vi "Pick modules.vi"(1 "Module List":T1(array[cluster])=[{"Enable"=TRUE, "Abs Start Time"=1500.0, "Module"=34, "String"="", "Array"=[]}, {"Enable"=FALSE, "Abs Start Time"=2000.0, "Module"=0, "String"="", "Array"=[]}, {"Enable"=FALSE, "Abs Start Time"=3000.0, "Module"=0, "String"="", "Array"=[]}, {"Enable"=FALSE, "Abs Start Time"=4000.0, "Module"=0, "String"="", "Array"=[]}, {"Enable"=TRUE, "Abs Start Time"=8000.0, "Module"=4, "String"="", "Array"=[]}, {"Enable"=FALSE, "Abs Start Time"=6000.0, "Module"=0, "String"="", "Array"=[]}] {"Module" items=["Atom removal 1", "Atom removal 2", "B-field off", "CMOT", "Defaults", "Final B-field ramps", "Fluorescence pulse", "High field", "High field ARP", "Loading cart QT", "Loading sci QT", "Low field", "Low field ARP", "Mol OD image", "Mol picture", "Mol probe pulse", "Molasses", "MOT off", "MOT on", "OD image", "Optical pumping", "OT B-field off", "Picture", "Probe pulse", "QT off for OT", "Quadrupole trap off", "Quadrupole trap", "Quantization axis", "S-G separation", "STIRAP back for imaging", "STIRAP", "TTL high", "TTL low", "GPIB", "Utility Module 1", "Utility Module 2", "Utility Module 3", "Utility Module 4", "Utility Module 5", "Utility Module 6", "Utility Module 7", "Utility Module 8", "Utility Module 9"]; "Abs Start Time" format="%.3f"}) -> (2 "Output Data":i64[][](array[numeric])=[[1600000, 3, 31, 1], [1600001, 3, 31, 0], [1700000, 3, 31, 1], [1700001, 3, 31, 0], [1800000, 3, 31, 1], [1800001, 3, 31, 0], [8000000, 0, 0, 0], [8000000, 0, 1, 0], [8000000, 0, 2, 0], [8000000, 0, 3, 0], [8000000, 0, 4, 1], [8000000, 0, 5, 0], [8000000, 0, 6, 0], [8000000, 0, 7, 0], [8000000, 0, 8, 0], [8000000, 0, 9, 1], [8000000, 0, 10, 0], [8000000, 0, 11, 0], [8000000, 0, 12, 0], [8000000, 0, 13, 0], [8000000, 0, 14, 1], [8000000, 0, 15, 0], [8000000, 0, 16, 0], [8000000, 0, 17, 0], [8000000, 0, 18, 0], [8000000, 0, 19, 1], [8000000, 0, 20, 0], [8000000, 0, 21, 0], [8000000, 0, 22, 0], [8000000, 0, 23, 0], [8000000, 0, 24, 1], [8000000, 0, 25, 0], [8000000, 0, 26, 0], [8000000, 0, 27, 0], [8000000, 0, 28, 0], [8000000, 0, 29, 0], [8000000, 0, 30, 0], [8000000, 0, 31, 0], [8000000, 1, 0, 0], [8000000, 1, 1, 0], [8000000, 1, 2, 0], [8000000, 1, 3, 0], [8000000, 1, 4, 0], [8000000, 1, 5, 0], [8000000, 1, 6, 0], [8000000, 1, 7, 0], [8000000, 1, 8, 0], [8000000, 1, 9, 0], [8000000, 1, 10, 0], [8000000, 1, 11, 0], [8000000, 1, 12, 0], [8000000, 1, 13, 0], [8000000, 1, 14, 0], [8000000, 1, 15, 0], [8000000, 1, 16, 0], [8000000, 1, 17, 1], [8000000, 1, 18, 0], [8000000, 1, 19, 0], [8000000, 1, 20, 0], [8000000, 1, 21, 0], [8000000, 1, 22, 0], [8000000, 1, 23, 0], [8000000, 1, 24, 0], [8000000, 1, 25, 0], [8000000, 1, 26, 0], [8000000, 1, 27, 0], [8000000, 1, 28, 0], [8000000, 1, 29, 0], [8000000, 1, 30, 0], [8000000, 1, 31, 0], [8000000, 2, 0, 0], [8000000, 2, 1, 0], [8000000, 2, 2, 0], [8000000, 2, 3, 0], [8000000, 2, 4, 0], [8000000, 2, 5, 0], [8000000, 2, 6, 0], [8000000, 2, 7, 0], [8000000, 2, 8, 0], [8000000, 2, 9, 0], [8000000, 2, 10, 0], [8000000, 2, 11, 0], [8000000, 2, 12, 0], [8000000, 2, 13, 0], [8000000, 2, 14, 0], [8000000, 2, 15, 0], [8000000, 2, 16, 0], [8000000, 2, 17, 0], [8000000, 2, 18, 0], [8000000, 2, 19, 0], [8000000, 2, 20, 0], [8000000, 2, 21, 0], [8000000, 2, 22, 0], [8000000, 2, 23, 0], [8000000, 2, 24, 0], [8000000, 2, 25, 0], [8000000, 2, 26, 0], [8000000, 2, 27, 0], [8000000, 2, 28, 0], [8000000, 2, 29, 0], [8000000, 2, 30, 0], [8000000, 2, 31, 0], [8000000, 3, 0, 0], [8000000, 3, 1, 0], [8000000, 3, 2, 0], [8000000, 3, 3, 0], [8000000, 3, 4, 0], [8000000, 3, 5, 0], [8000000, 3, 6, 0], [8000000, 3, 7, 0], [8000000, 3, 8, 0], [8000000, 3, 9, 0], [8000000, 3, 10, 0], [8000000, 3, 11, 0], [8000000, 3, 12, 0], [8000000, 3, 13, 0], [8000000, 3, 14, 0], [8000000, 3, 15, 0], [8000000, 3, 16, 0], [8000000, 3, 17, 0], [8000000, 3, 18, 0], [8000000, 3, 19, 0], [8000000, 3, 20, 0], [8000000, 3, 21, 0], [8000000, 3, 22, 0], [8000000, 3, 23, 0], [8000000, 3, 24, 0], [8000000, 3, 25, 0], [8000000, 3, 26, 0], [8000000, 3, 27, 0], [8000000, 3, 28, 0], [8000000, 3, 29, 0], [8000000, 3, 30, 0], [8000000, 3, 31, 0]], 3 "GPIB output":T1(array[cluster]) {"Module" items=["TTL high                                                                                 ", "TTL low                          ", "Camera Strobe                   ", "Defaults                           ", "Fluorescence pulse           ", "IP trap                         ", "Kinetics OD image          ", "MOT light only                ", "MOT off                                   ", "MOT on                         ", "Move cart                      ", "OD image                     ", "Optical pumping          ", "Picture                             ", "Quadrupole trap             ", "Utility Module 01          ", "Utility Module 02           ", "Utility Module 03           ", "Utility Module 04           ", "CMOT", "Static DAQ", "GPIB"]; "Abs Start Time" format="%.3f"}, 4 "Static output":T2(array[cluster])=[{"Times"=[], "Voltages"=[], "Enable Ch"=TRUE, "Hinge Points"=0}, {"Times"=[], "Voltages"=[], "Enable Ch"=TRUE, "Hinge Points"=0}, {"Times"=[], "Voltages"=[], "Enable Ch"=TRUE, "Hinge Points"=0}, {"Times"=[], "Voltages"=[], "Enable Ch"=TRUE, "Hinge Points"=0}, {"Times"=[], "Voltages"=[], "Enable Ch"=TRUE, "Hinge Points"=0}, {"Times"=[], "Voltages"=[], "Enable Ch"=TRUE, "Hinge Points"=0}, {"Times"=[], "Voltages"=[], "Enable Ch"=TRUE, "Hinge Points"=0}, {"Times"=[], "Voltages"=[], "Enable Ch"=TRUE, "Hinge Points"=0}, {"Times"=[], "Voltages"=[], "Enable Ch"=TRUE, "Hinge Points"=0}, {"Times"=[], "Voltages"=[], "Enable Ch"=TRUE, "Hinge Points"=0}, {"Times"=[], "Voltages"=[], "Enable Ch"=TRUE, "Hinge Points"=0}, {"Times"=[], "Voltages"=[], "Enable Ch"=TRUE, "Hinge Points"=0}, {"Times"=[], "Voltages"=[], "Enable Ch"=TRUE, "Hinge Points"=0}, {"Times"=[], "Voltages"=[], "Enable Ch"=TRUE, "Hinge Points"=0}, {"Times"=[], "Voltages"=[], "Enable Ch"=TRUE, "Hinge Points"=0}, {"Times"=[], "Voltages"=[], "Enable Ch"=TRUE, "Hinge Points"=0}] {"Voltages" format="%.2f"; "Times" format="%.2f"})   [LabVIEW 2017]
doc: "This subVI goes through the module list, picks the right subVIs, and adds the their TTL actions to the Input Array. This module also adds TTL pulses for setting the initial and final Static DAC values.\n The outputs of this vi are 3 arrays: for the TTL stuff, the Static DACS, and the GPIB commands."
uses:
  globals/Modules global.vi
panel:
  out "GPIB temp":T1(array[cluster]) {"Module" items=["TTL high                                                                                 ", "TTL low                          ", "Camera Strobe                   ", "Defaults                           ", "Fluorescence pulse           ", "IP trap                         ", "Kinetics OD image          ", "MOT light only                ", "MOT off                                   ", "MOT on                         ", "Move cart                      ", "OD image                     ", "Optical pumping          ", "Picture                             ", "Quadrupole trap             ", "Utility Module 01          ", "Utility Module 02           ", "Utility Module 03           ", "Utility Module 04           ", "CMOT", "Static DAQ", "GPIB"]; "Abs Start Time" format="%.3f"}
  out "Static temp":T2(array[cluster])=[{"Times"=[], "Voltages"=[], "Enable Ch"=TRUE, "Hinge Points"=0}, {"Times"=[], "Voltages"=[], "Enable Ch"=TRUE, "Hinge Points"=0}, {"Times"=[], "Voltages"=[], "Enable Ch"=TRUE, "Hinge Points"=0}, {"Times"=[], "Voltages"=[], "Enable Ch"=TRUE, "Hinge Points"=0}, {"Times"=[], "Voltages"=[], "Enable Ch"=TRUE, "Hinge Points"=0}, {"Times"=[], "Voltages"=[], "Enable Ch"=TRUE, "Hinge Points"=0}, {"Times"=[], "Voltages"=[], "Enable Ch"=TRUE, "Hinge Points"=0}, {"Times"=[], "Voltages"=[], "Enable Ch"=TRUE, "Hinge Points"=0}, {"Times"=[], "Voltages"=[], "Enable Ch"=TRUE, "Hinge Points"=0}, {"Times"=[], "Voltages"=[], "Enable Ch"=TRUE, "Hinge Points"=0}, {"Times"=[], "Voltages"=[], "Enable Ch"=TRUE, "Hinge Points"=0}, {"Times"=[], "Voltages"=[], "Enable Ch"=TRUE, "Hinge Points"=0}, {"Times"=[], "Voltages"=[], "Enable Ch"=TRUE, "Hinge Points"=0}, {"Times"=[], "Voltages"=[], "Enable Ch"=TRUE, "Hinge Points"=0}, {"Times"=[], "Voltages"=[], "Enable Ch"=TRUE, "Hinge Points"=0}, {"Times"=[], "Voltages"=[], "Enable Ch"=TRUE, "Hinge Points"=0}] {"Voltages" format="%.2f"; "Times" format="%.2f"}
  out "Numeric":dbl=5.0 format="%.2f"
  out "Temp":i64[][](array[numeric])=[[1600000, 3, 31, 1], [1600001, 3, 31, 0], [1700000, 3, 31, 1], [1700001, 3, 31, 0], [1800000, 3, 31, 1], [1800001, 3, 31, 0], [8000000, 0, 0, 0], [8000000, 0, 1, 0], [8000000, 0, 2, 0], [8000000, 0, 3, 0], [8000000, 0, 4, 1], [8000000, 0, 5, 0], [8000000, 0, 6, 0], [8000000, 0, 7, 0], [8000000, 0, 8, 0], [8000000, 0, 9, 1], [8000000, 0, 10, 0], [8000000, 0, 11, 0], [8000000, 0, 12, 0], [8000000, 0, 13, 0], [8000000, 0, 14, 1], [8000000, 0, 15, 0], [8000000, 0, 16, 0], [8000000, 0, 17, 0], [8000000, 0, 18, 0], [8000000, 0, 19, 1], [8000000, 0, 20, 0], [8000000, 0, 21, 0], [8000000, 0, 22, 0], [8000000, 0, 23, 0], [8000000, 0, 24, 1], [8000000, 0, 25, 0], [8000000, 0, 26, 0], [8000000, 0, 27, 0], [8000000, 0, 28, 0], [8000000, 0, 29, 0], [8000000, 0, 30, 0], [8000000, 0, 31, 0], [8000000, 1, 0, 0], [8000000, 1, 1, 0], [8000000, 1, 2, 0], [8000000, 1, 3, 0], [8000000, 1, 4, 0], [8000000, 1, 5, 0], [8000000, 1, 6, 0], [8000000, 1, 7, 0], [8000000, 1, 8, 0], [8000000, 1, 9, 0], [8000000, 1, 10, 0], [8000000, 1, 11, 0], [8000000, 1, 12, 0], [8000000, 1, 13, 0], [8000000, 1, 14, 0], [8000000, 1, 15, 0], [8000000, 1, 16, 0], [8000000, 1, 17, 1], [8000000, 1, 18, 0], [8000000, 1, 19, 0], [8000000, 1, 20, 0], [8000000, 1, 21, 0], [8000000, 1, 22, 0], [8000000, 1, 23, 0], [8000000, 1, 24, 0], [8000000, 1, 25, 0], [8000000, 1, 26, 0], [8000000, 1, 27, 0], [8000000, 1, 28, 0], [8000000, 1, 29, 0], [8000000, 1, 30, 0], [8000000, 1, 31, 0], [8000000, 2, 0, 0], [8000000, 2, 1, 0], [8000000, 2, 2, 0], [8000000, 2, 3, 0], [8000000, 2, 4, 0], [8000000, 2, 5, 0], [8000000, 2, 6, 0], [8000000, 2, 7, 0], [8000000, 2, 8, 0], [8000000, 2, 9, 0], [8000000, 2, 10, 0], [8000000, 2, 11, 0], [8000000, 2, 12, 0], [8000000, 2, 13, 0], [8000000, 2, 14, 0], [8000000, 2, 15, 0], [8000000, 2, 16, 0], [8000000, 2, 17, 0], [8000000, 2, 18, 0], [8000000, 2, 19, 0], [8000000, 2, 20, 0], [8000000, 2, 21, 0], [8000000, 2, 22, 0], [8000000, 2, 23, 0], [8000000, 2, 24, 0], [8000000, 2, 25, 0], [8000000, 2, 26, 0], [8000000, 2, 27, 0], [8000000, 2, 28, 0], [8000000, 2, 29, 0], [8000000, 2, 30, 0], [8000000, 2, 31, 0], [8000000, 3, 0, 0], [8000000, 3, 1, 0], [8000000, 3, 2, 0], [8000000, 3, 3, 0], [8000000, 3, 4, 0], [8000000, 3, 5, 0], [8000000, 3, 6, 0], [8000000, 3, 7, 0], [8000000, 3, 8, 0], [8000000, 3, 9, 0], [8000000, 3, 10, 0], [8000000, 3, 11, 0], [8000000, 3, 12, 0], [8000000, 3, 13, 0], [8000000, 3, 14, 0], [8000000, 3, 15, 0], [8000000, 3, 16, 0], [8000000, 3, 17, 0], [8000000, 3, 18, 0], [8000000, 3, 19, 0], [8000000, 3, 20, 0], [8000000, 3, 21, 0], [8000000, 3, 22, 0], [8000000, 3, 23, 0], [8000000, 3, 24, 0], [8000000, 3, 25, 0], [8000000, 3, 26, 0], [8000000, 3, 27, 0], [8000000, 3, 28, 0], [8000000, 3, 29, 0], [8000000, 3, 30, 0], [8000000, 3, 31, 0]]
  # "Input and Output arrays are time (board units), port, line, value."
  # "Enable  Time         Module                    Parameters                  Comments  \n                                                        (port A-D)  (line 0-15)"
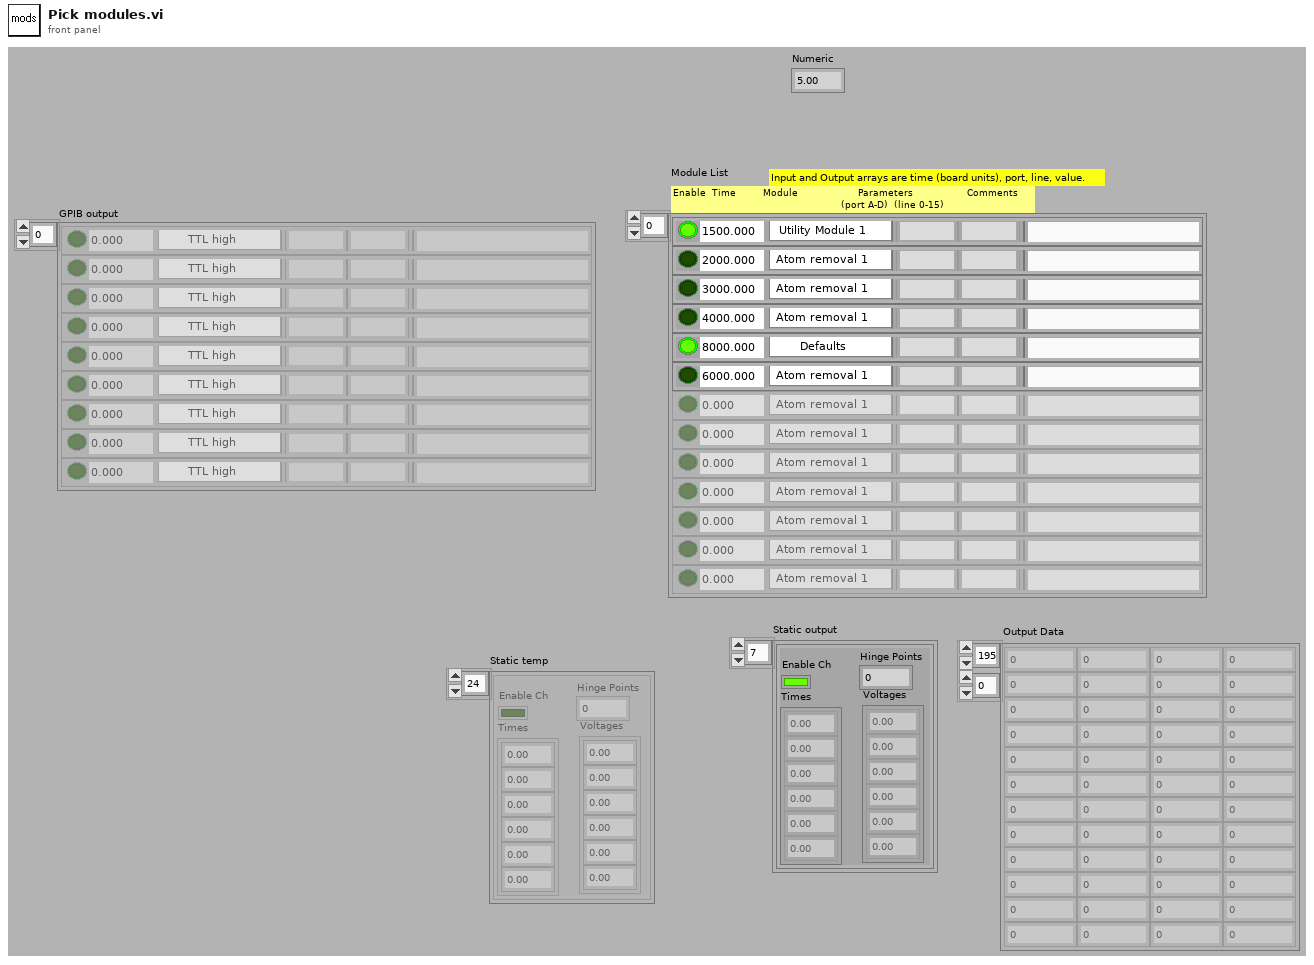
[diagram p1: front panel]
types:
  T1 = cluster{"Enable":bool, "Abs Start Time":dbl, "Module":u16, "String":string, "Array":string[]}[]
  T2 = cluster{"Times":dbl[], "Voltages":dbl[], "Enable Ch":bool, "Hinge Points":u8}[]
  T3 = cluster{"Enable":bool, "Abs Start Time":dbl, "Module":u16, "String":string, "Array":string[]}
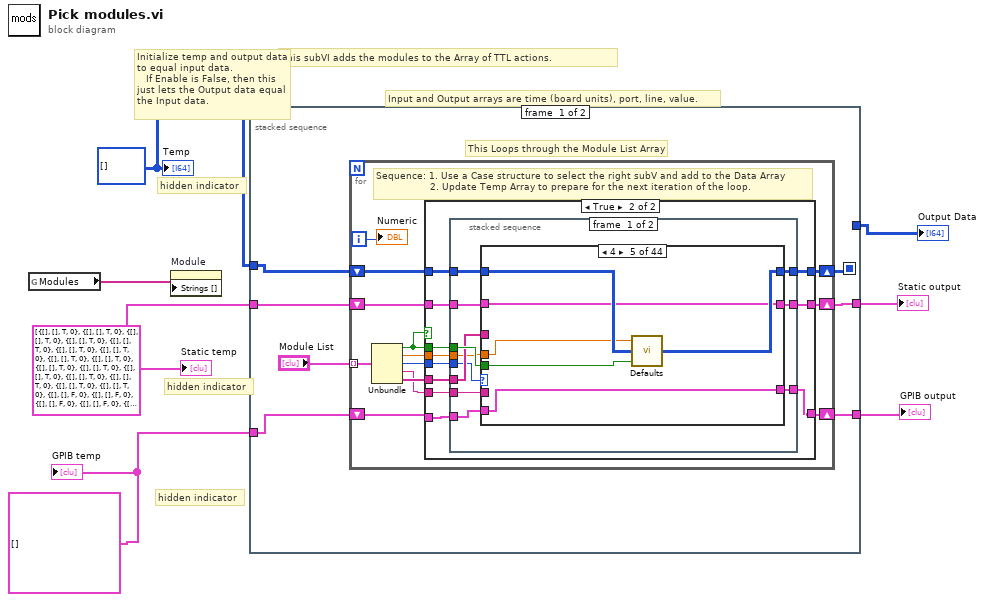
[diagram p0: block diagram]
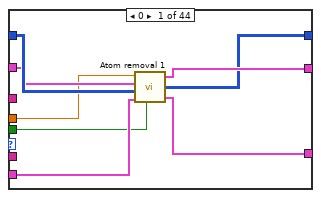
[diagram p3: hidden frame]
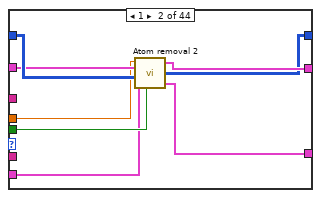
[diagram p4: hidden frame]
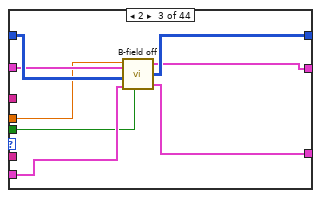
[diagram p5: hidden frame]
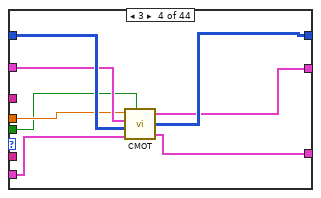
[diagram p6: hidden frame]
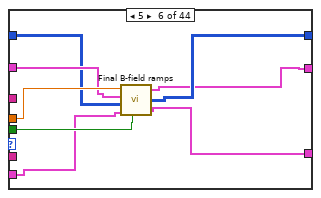
[diagram p7: hidden frame]
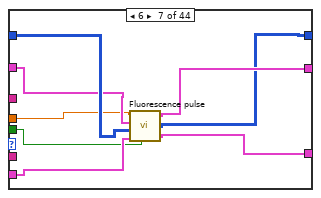
[diagram p8: hidden frame]
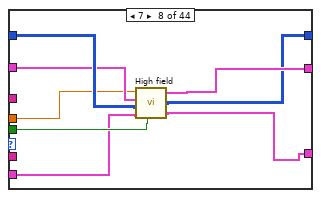
[diagram p9: hidden frame]
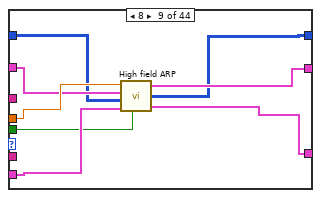
[diagram p10: hidden frame]
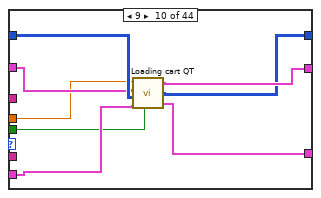
[diagram p11: hidden frame]
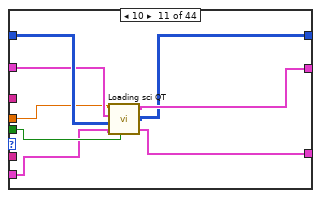
[diagram p12: hidden frame]
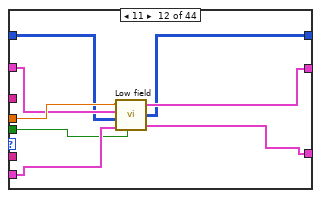
[diagram p13: hidden frame]
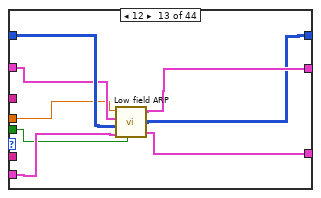
[diagram p14: hidden frame]
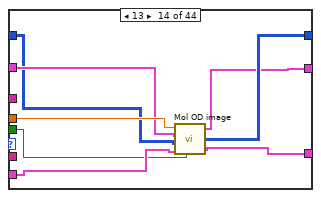
[diagram p15: hidden frame]
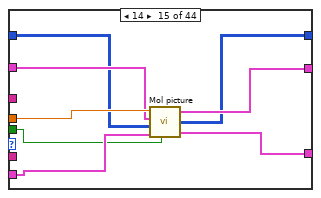
[diagram p16: hidden frame]
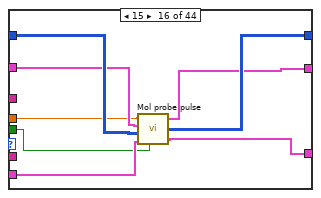
[diagram p17: hidden frame]
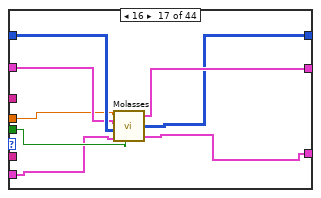
[diagram p18: hidden frame]
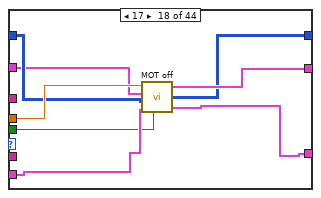
[diagram p19: hidden frame]
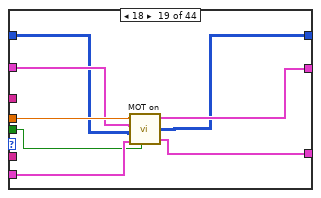
[diagram p20: hidden frame]
diagram:
  w4 = T1 [] ("GPIB output")
  w7 = T2 [{"Times"=[], "Voltages"=[], "Enable Ch"=TRUE, "Hinge Points"=0}, {"Times"=[], "Voltages"=[], "Enable Ch"=TRUE, "Hinge Points"=0}, {"Times"=[], "Voltages"=[], "Enable Ch"=TRUE, "Hinge Points"=0}, {"Times"=[], "Voltages"=[], "Enable Ch"=TRUE, "Hinge Points"=0}, {"Times"=[], "Voltages"=[], "Enable Ch"=TRUE, "Hinge Points"=0}, {"Times"=[], "Voltages"=[], "Enable Ch"=TRUE, "Hinge Points"=0}, {"Times"=[], "Voltages"=[], "Enable Ch"=TRUE, "Hinge Points"=0}, {"Times"=[], "Voltages"=[], "Enable Ch"=TRUE, "Hinge Points"=0}, {"Times"=[], "Voltages"=[], "Enable Ch"=TRUE, "Hinge Points"=0}, {"Times"=[], "Voltages"=[], "Enable Ch"=TRUE, "Hinge Points"=0}, {"Times"=[], "Voltages"=[], "Enable Ch"=TRUE, "Hinge Points"=0}, {"Times"=[], "Voltages"=[], "Enable Ch"=TRUE, "Hinge Points"=0}, {"Times"=[], "Voltages"=[], "Enable Ch"=TRUE, "Hinge Points"=0}, {"Times"=[], "Voltages"=[], "Enable Ch"=TRUE, "Hinge Points"=0}, {"Times"=[], "Voltages"=[], "Enable Ch"=TRUE, "Hinge Points"=0}, {"Times"=[], "Voltages"=[], "Enable Ch"=TRUE, "Hinge Points"=0}, {"Times"=[], "Voltages"=[], "Enable Ch"=FALSE, "Hinge Points"=0}, {"Times"=[], "Voltages"=[], "Enable Ch"=FALSE, "Hinge Points"=0}, {"Times"=[], "Voltages"=[], "Enable Ch"=FALSE, "Hinge Points"=0}, {"Times"=[], "Voltages"=[], "Enable Ch"=FALSE, "Hinge Points"=0}, {"Times"=[], "Voltages"=[], "Enable Ch"=FALSE, "Hinge Points"=0}, {"Times"=[], "Voltages"=[], "Enable Ch"=FALSE, "Hinge Points"=0}, {"Times"=[], "Voltages"=[], "Enable Ch"=FALSE, "Hinge Points"=0}, {"Times"=[], "Voltages"=[], "Enable Ch"=TRUE, "Hinge Points"=0}] ("Array")
  w6 = i64[][] [] ("Sorted array 2")
  # "hidden indicator"
  # "hidden indicator"
  # "Input and Output arrays are time (board units), port, line, value."
  # "This subVI adds the modules to the Array of TTL actions."
  # "hidden indicator"
  n1 = global read "Modules global.vi" "Modules"() -> (w2:string[])
  n2 = property on="Module" class="Ring (strict)"("Strings []"=w2) -> ()  [unwired: 2 in, 2 out]
  n3 = stacked-sequence {
    seq-local: [w11 _] -> [_ w413]
    tunnel: w7 -> [w13 _]
    tunnel: w6 -> [w12 _]
    tunnel: [w10 _] -> w5
    tunnel: w4 -> [w8 _]
    tunnel: [w9 _] -> w3
    tunnel: [_ w413] -> w1
    frame #0 {
      # "This Loops through the Module List Array"
      # "Initialize temp and output data to equal input data. \n   If Enable is False, then this just lets the Output data equal the Input data."
      n4 = for {
        tunnel: "Module List" -> [w22] mode=indexing
        shift-right: [w17] -> w11
        shift-left: w12 -> [w18]
        shift-right: [w19] -> w10
        shift-left: w13 -> [w20]
        shift-right: [w15] -> w9
        shift-left: w8 -> [w16]
        i -> [w24]
        # "Sequence: 1. Use a Case structure to select the right subV and add to the Data Array\n                  2. Update Temp Array to prepare for the next iteration of the loop."
        n5 = Unbundle(w22) -> ("Enable"=w23:bool, "Abs Start Time"=w26:dbl, "Module"=w27:u16, "String"=w21:string, "Array"=w25:string[])
        n6 = case shown="True" w23 {
          tunnel: w23 -> [_ w38]
          tunnel: w27 -> [_ w41]
          tunnel: w26 -> [_ w40]
          tunnel: w25 -> [_ w39]
          tunnel: w21 -> [_ w37]
          tunnel: w20 -> [w29 w36]
          tunnel: [w29 w35] -> w19
          tunnel: w18 -> [w30 w34]
          tunnel: [w30 w33] -> w17
          tunnel: w16 -> [w28 w32]
          tunnel: [w28 w31] -> w15
          frame False {
          }
          frame True {
            n7 = stacked-sequence {
              tunnel: w38 -> [w52 _]
              tunnel: w41 -> [w50 _]
              tunnel: w40 -> [w49 _]
              tunnel: w39 -> [w51 _]
              tunnel: w37 -> [w48 _]
              tunnel: w36 -> [w47 _]
              tunnel: [w46 _] -> w35
              tunnel: w34 -> [w45 _]
              tunnel: [w44 _] -> w33
              tunnel: w32 -> [w43 _]
              tunnel: [w42 _] -> w31
              frame #0 {
                n8 = case shown="4" w50 {
                  selector: w50 -> [_ _ _ _ _ _ _ _ _ _ _ _ _ _ _ _ _ _ _ _ _ _ _ _ _ _ _ _ _ _ _ _ _ w333 _ _ _ _ _ _ _ _ _ _]
                  tunnel: w52 -> [w54 w65 w70 w77 w90 w94 w99 w111 w115 w123 w135 w139 w150 w158 w163 w171 w183 w187 w195 w206 w211 w219 w227 w235 w246 w255 w259 w267 w275 w286 w294 w310 w314 w331 w335 w343 w351 w359 w367 w375 w383 w391 w399 _]
                  tunnel: w51 -> [_ _ _ _ _ _ _ _ _ _ _ _ _ _ _ _ _ _ _ _ _ _ _ _ _ _ _ _ _ _ _ w306 w312 w328 _ _ _ _ _ _ _ _ _ _]
                  tunnel: w49 -> [w53 w66 w69 w78 w88 w95 w100 w107 w119 w124 w131 w143 w147 w162 w167 w172 w179 w191 w199 w210 w215 w220 w231 w239 w244 w251 w260 w271 w279 w287 w293 w299 w313 w330 w336 w344 w355 w360 w368 w379 w384 w395 w400 _]
                  tunnel: w48 -> [_ _ _ _ _ _ _ _ _ _ _ _ _ _ _ _ _ _ _ _ _ _ _ _ _ _ _ _ _ _ _ _ _ w332 _ _ _ _ _ _ _ _ _ _]
                  tunnel: w47 -> [w59 w67 w75 w79 w86 w93 w101 w108 w118 w125 w132 w142 w148 w161 w166 w173 w180 w189 w198 w209 w214 w221 w230 w238 w245 w252 w261 w268 w278 w283 w291 w307 w320 w325 w337 w345 w354 w361 w369 w378 w385 w394 w401 w408]
                  tunnel: [w57 w64 w71 w83 w86 w96 w106 w114 w122 w130 w138 w146 w154 w156 w170 w177 w186 w194 w202 w205 w218 w226 w234 w242 w250 w258 w266 w274 w282 w290 w295 w307 w320 w325 w342 w350 w358 w366 w374 w382 w390 w398 w406 w408] -> w46
                  tunnel: w45 -> [w60 w68 w76 w80 w89 w92 w102 w109 w117 w126 w133 w141 w149 w160 w165 w174 w181 w190 w197 w208 w213 w222 w229 w237 w243 w253 w262 w269 w277 w284 w292 w309 w316 w326 w338 w346 w353 w362 w370 w377 w386 w393 w402 w409]
                  tunnel: [w56 w63 w72 w84 w87 w97 w105 w113 w121 w129 w137 w145 w153 w157 w169 w178 w185 w193 w201 w204 w217 w225 w233 w241 w249 w257 w265 w273 w281 w289 w296 w308 w315 w326 w341 w349 w357 w365 w373 w381 w389 w397 w405 w409] -> w44
                  tunnel: w43 -> [w58 w61 w74 w81 w85 w91 w103 w110 w116 w127 w134 w140 w151 w159 w164 w175 w182 w188 w196 w207 w212 w223 w228 w236 w247 w254 w263 w270 w276 w285 w298 w311 w319 w329 w339 w347 w352 w363 w371 w376 w387 w392 w403 w407]
                  tunnel: [w55 w62 w73 w82 w85 w98 w104 w112 w120 w128 w136 w144 w152 w155 w168 w176 w184 w192 w200 w203 w216 w224 w232 w240 w248 w256 w264 w272 w280 w288 w297 w311 w319 w327 w340 w348 w356 w364 w372 w380 w388 w396 w404 w407] -> w42
                  frame 0 {
                    n9 = call "Atom removal 1.vi"("Absolute start time (ms)"=w53, "Static input"=w59, "Input"=w60, "GPIB Input"=w58, "Do this?"=w54) -> ("Static output"=w57:T2, "Output"=w56:i64[][], "GPIB Output"=w55:T1)
                  }
                  frame 1 {
                    n10 = call "Atom removal 2.vi"("Absolute start time (ms)"=w66, "Static input"=w67, "Input"=w68, "GPIB Input"=w61, "Do this?"=w65) -> ("Static output"=w64:T2, "Output"=w63:i64[][], "GPIB Output"=w62:T1)
                  }
                  frame 2 {
                    n11 = call "B-field off.vi"("Absolute start time (ms)"=w69, "Static input"=w75, "Input"=w76, "GPIB Input"=w74, "Do this?"=w70) -> ("Static output"=w71:T2, "Output"=w72:i64[][], "GPIB Output"=w73:T1)
                  }
                  frame 3 {
                    n12 = call "CMOT.vi"("Absolute start time (ms)"=w78, "Static input"=w79, "Input"=w80, "GPIB Input"=w81, "Do this?"=w77) -> ("Static output"=w83:T2, "Output"=w84:i64[][], "GPIB Output"=w82:T1)
                  }
                  frame 4 {
                    n13 = call "Defaults.vi"("Do this?"=w90, "Input"=w89, "Absolute start time (ms)"=w88) -> ("Output"=w87:i64[][])
                  }
                  frame 5 {
                    n14 = call "Final B-field ramps.vi"("Absolute start time (ms)"=w95, "Static input"=w93, "Input"=w92, "GPIB Input"=w91, "Do this?"=w94) -> ("Static output"=w96:T2, "Output"=w97:i64[][], "GPIB Output"=w98:T1)
                  }
                  frame 6 {
                    n15 = call "Fluorescence pulse.vi"("Absolute start time (ms)"=w100, "Static input"=w101, "Input"=w102, "GPIB Input"=w103, "Do this?"=w99) -> ("Static output"=w106:T2, "Output"=w105:i64[][], "GPIB Output"=w104:T1)
                  }
                  frame 7 {
                    n16 = call "High field.vi"("Absolute start time (ms)"=w107, "Static input"=w108, "Input"=w109, "GPIB Input"=w110, "Do this?"=w111) -> ("Static output"=w114:T2, "Output"=w113:i64[][], "GPIB Output"=w112:T1)
                  }
                  frame 8 {
                    n17 = call "High field ARP.vi"("Absolute start time (ms)"=w119, "Static input"=w118, "Input"=w117, "GPIB Input"=w116, "Do this?"=w115) -> ("Static output"=w122:T2, "Output"=w121:i64[][], "GPIB Output"=w120:T1)
                  }
                  frame 9 {
                    n18 = call "Loading cart QT.vi"("Absolute start time (ms)"=w124, "Static input"=w125, "Input"=w126, "GPIB Input"=w127, "Do this?"=w123) -> ("Static output"=w130:T2, "Output"=w129:i64[][], "GPIB Output"=w128:T1)
                  }
                  frame 10 {
                    n19 = call "Loading sci QT.vi"("Absolute start time (ms)"=w131, "Static input"=w132, "Input"=w133, "GPIB Input"=w134, "Do this?"=w135) -> ("Static output"=w138:T2, "Output"=w137:i64[][], "GPIB Output"=w136:T1)
                  }
                  frame 11 {
                    n20 = call "Low field.vi"("Absolute start time (ms)"=w143, "Static input"=w142, "Input"=w141, "GPIB Input"=w140, "Do this?"=w139) -> ("Static output"=w146:T2, "Output"=w145:i64[][], "GPIB Output"=w144:T1)
                  }
                  frame 12 {
                    n21 = call "Low field ARP.vi"("Absolute start time (ms)"=w147, "Static input"=w148, "Input"=w149, "GPIB Input"=w151, "Do this?"=w150) -> ("Static output"=w154:T2, "Output"=w153:i64[][], "GPIB Output"=w152:T1)
                  }
                  frame 13 {
                    n22 = call "Mol OD image.vi"("Absolute start time (ms)"=w162, "Static input"=w161, "Input"=w160, "GPIB Input"=w159, "Do this?"=w158) -> ("Static output"=w156:T2, "Output"=w157:i64[][], "GPIB Output"=w155:T1)
                  }
                  frame 14 {
                    n23 = call "Mol picture.vi"("Absolute start time (ms)"=w167, "Static input"=w166, "Input"=w165, "GPIB Input"=w164, "Do this?"=w163) -> ("Static output"=w170:T2, "Output"=w169:i64[][], "GPIB Output"=w168:T1)
                  }
                  frame 15 {
                    n24 = call "Mol probe pulse.vi"("Absolute start time (ms)"=w172, "Static input"=w173, "Input"=w174, "GPIB Input"=w175, "Do this?"=w171) -> ("Static output"=w177:T2, "Output"=w178:i64[][], "GPIB Output"=w176:T1)
                  }
                  frame 16 {
                    n25 = call "Molasses.vi"("Absolute start time (ms)"=w179, "Static input"=w180, "Input"=w181, "GPIB Input"=w182, "Do this?"=w183) -> ("Static output"=w186:T2, "Output"=w185:i64[][], "GPIB Output"=w184:T1)
                  }
                  frame 17 {
                    n26 = call "MOT off.vi"("Absolute start time (ms)"=w191, "Static input"=w189, "Input"=w190, "GPIB Input"=w188, "Do this?"=w187) -> ("Static output"=w194:T2, "Output"=w193:i64[][], "GPIB Output"=w192:T1)
                  }
                  frame 18 {
                    n27 = call "MOT on.vi"("Absolute start time (ms)"=w199, "Static input"=w198, "Input"=w197, "GPIB Input"=w196, "Do this?"=w195) -> ("Static output"=w202:T2, "Output"=w201:i64[][], "GPIB Output"=w200:T1)
                  }
                  frame 19 {
                    n28 = call "OD image.vi"("Absolute start time (ms)"=w210, "Static input"=w209, "Input"=w208, "GPIB Input"=w207, "Do this?"=w206) -> ("Static output"=w205:T2, "Output"=w204:i64[][], "GPIB Output"=w203:T1)
                  }
                  frame 20 {
                    n29 = call "Optical pumping.vi"("Absolute start time (ms)"=w215, "Static input"=w214, "Input"=w213, "GPIB Input"=w212, "Do this?"=w211) -> ("Static output"=w218:T2, "Output"=w217:i64[][], "GPIB Output"=w216:T1)
                  }
                  frame 21 {
                    n30 = call "OT B-field off.vi"("Absolute start time (ms)"=w220, "Static input"=w221, "Input"=w222, "GPIB Input"=w223, "Do this?"=w219) -> ("Static output"=w226:T2, "Output"=w225:i64[][], "GPIB Output"=w224:T1)
                  }
                  frame 22 {
                    n31 = call "Picture.vi"("Absolute start time (ms)"=w231, "Static input"=w230, "Input"=w229, "GPIB Input"=w228, "Do this?"=w227) -> ("Static output"=w234:T2, "Output"=w233:i64[][], "GPIB Output"=w232:T1)
                  }
                  frame 23 {
                    n32 = call "Probe pulse.vi"("Absolute start time (ms)"=w239, "Static input"=w238, "Input"=w237, "GPIB Input"=w236, "Do this?"=w235) -> ("Static output"=w242:T2, "Output"=w241:i64[][], "GPIB Output"=w240:T1)
                  }
                  frame 24 {
                    n33 = call "QT off for OT.vi"("Absolute start time (ms)"=w244, "Static input"=w245, "Input"=w243, "GPIB Input"=w247, "Do this?"=w246) -> ("Static output"=w250:T2, "Output"=w249:i64[][], "GPIB Output"=w248:T1)
                  }
                  frame 25 {
                    n34 = call "Quadrupole trap off.vi"("Absolute start time (ms)"=w251, "Static input"=w252, "Input"=w253, "GPIB Input"=w254, "Do this?"=w255) -> ("Static output"=w258:T2, "Output"=w257:i64[][], "GPIB Output"=w256:T1)
                  }
                  frame 26 {
                    n35 = call "Quadrupole trap.vi"("Absolute start time (ms)"=w260, "Static input"=w261, "Input"=w262, "GPIB Input"=w263, "Do this?"=w259) -> ("Static output"=w266:T2, "Output"=w265:i64[][], "GPIB Output"=w264:T1)
                  }
                  frame 27 {
                    n36 = call "Quantization axis.vi"("Absolute start time (ms)"=w271, "Static input"=w268, "Input"=w269, "GPIB Input"=w270, "Do this?"=w267) -> ("Static output"=w274:T2, "Output"=w273:i64[][], "GPIB Output"=w272:T1)
                  }
                  frame 28 {
                    n37 = call "S-G separation.vi"("Absolute start time (ms)"=w279, "Static input"=w278, "Input"=w277, "GPIB Input"=w276, "Do this?"=w275) -> ("Static output"=w282:T2, "Output"=w281:i64[][], "GPIB Output"=w280:T1)
                  }
                  frame 29 {
                    n38 = call "STIRAP back for imaging.vi"("Absolute start time (ms)"=w287, "Static input"=w283, "Input"=w284, "GPIB Input"=w285, "Do this?"=w286) -> ("Static output"=w290:T2, "Output"=w289:i64[][], "GPIB Output"=w288:T1)
                  }
                  frame 30 {
                    n39 = call "STIRAP.vi"("Absolute start time (ms)"=w293, "Static input"=w291, "Input"=w292, "GPIB Input"=w298, "Do this?"=w294) -> ("Static output"=w295:T2, "Output"=w296:i64[][], "GPIB Output"=w297:T1)
                  }
                  frame 31 {
                    n40 = Index Array(array=w306) -> (element #1=w303:string, element #2=w305:string)  [unwired: 2 in]
                    n41 = Hexadecimal String To Number(string=w303) -> (number=w302:u32)  [unwired: 2 in, 1 out]
                    n42 = Subtract(x=w302, y=u32 10) -> (x-y=w300:u32)
                    n43 = Decimal String To Number(string=w305) -> (number=w304:i32)  [unwired: 2 in, 1 out]
                    n44 = call "TTL high.vi"("Line"=w304, "Port"=w300, "Do this?"=w310, "Input"=w309, "Absolute start time (ms)"=w299) -> ("Output"=w308:i64[][])
                  }
                  frame 32 {
                    n45 = Index Array(array=w312) -> (element #1=w323:string, element #2=w324:string)  [unwired: 2 in]
                    n46 = Hexadecimal String To Number(string=w323) -> (number=w322:u32)  [unwired: 2 in, 1 out]
                    n47 = Subtract(x=w322, y=u32 10) -> (x-y=w318:u32)
                    n48 = Decimal String To Number(string=w324) -> (number=w317:i32)  [unwired: 2 in, 1 out]
                    n49 = call "TTL low.vi"("Line"=w317, "Port"=w318, "Do this?"=w314, "Input"=w316, "Absolute start time (ms)"=w313) -> ("Output"=w315:i64[][])
                  }
                  frame 33 {
                    n50 = Bundle("Enable"=w331, "Abs Start Time"=w330, "Module"=w333, "String"=w332, "Array"=w328) -> (w334:T3)  [unwired: 1 in]
                    n51 = Build Array (concatenate)(w329, w334) -> (w327:T1)
                  }
                  frame 34 {
                    n52 = call "Utility Module 1.vi"("Absolute start time (ms)"=w336, "Static input"=w337, "Input"=w338, "GPIB Input"=w339, "Do this?"=w335) -> ("Static output"=w342:T2, "Output"=w341:i64[][], "GPIB Output"=w340:T1)
                  }
                  frame 35 {
                    n53 = call "Utility Module 2.vi"("Absolute start time (ms)"=w344, "Static input"=w345, "Input"=w346, "GPIB Input"=w347, "Do this?"=w343) -> ("Static output"=w350:T2, "Output"=w349:i64[][], "GPIB Output"=w348:T1)
                  }
                  frame 36 {
                    n54 = call "Utility Module 3.vi"("Absolute start time (ms)"=w355, "Static input"=w354, "Input"=w353, "GPIB Input"=w352, "Do this?"=w351) -> ("Static output"=w358:T2, "Output"=w357:i64[][], "GPIB Output"=w356:T1)
                  }
                  frame 37 {
                    n55 = call "Utility Module 4.vi"("Absolute start time (ms)"=w360, "Static input"=w361, "Input"=w362, "GPIB Input"=w363, "Do this?"=w359) -> ("Static output"=w366:T2, "Output"=w365:i64[][], "GPIB Output"=w364:T1)
                  }
                  frame 38 {
                    n56 = call "Utility Module 5.vi"("Absolute start time (ms)"=w368, "Static input"=w369, "Input"=w370, "GPIB Input"=w371, "Do this?"=w367) -> ("Static output"=w374:T2, "Output"=w373:i64[][], "GPIB Output"=w372:T1)
                  }
                  frame 39 {
                    n57 = call "Utility Module 6.vi"("Absolute start time (ms)"=w379, "Static input"=w378, "Input"=w377, "GPIB Input"=w376, "Do this?"=w375) -> ("Static output"=w382:T2, "Output"=w381:i64[][], "GPIB Output"=w380:T1)
                  }
                  frame 40 {
                    n58 = call "Utility Module 7.vi"("Absolute start time (ms)"=w384, "Static input"=w385, "Input"=w386, "GPIB Input"=w387, "Do this?"=w383) -> ("Static output"=w390:T2, "Output"=w389:i64[][], "GPIB Output"=w388:T1)
                  }
                  frame 41 {
                    n59 = call "Utility Module 8.vi"("Absolute start time (ms)"=w395, "Static input"=w394, "Input"=w393, "GPIB Input"=w392, "Do this?"=w391) -> ("Static output"=w398:T2, "Output"=w397:i64[][], "GPIB Output"=w396:T1)
                  }
                  frame 42 {
                    n60 = call "Utility Module 9.vi"("Absolute start time (ms)"=w400, "Static input"=w401, "Input"=w402, "GPIB Input"=w403, "Do this?"=w399) -> ("Static output"=w406:T2, "Output"=w405:i64[][], "GPIB Output"=w404:T1)
                  }
                  frame 43, Default {
                  }
                }
              }
              frame #1 {
                # "Update Temp array"
                n61 = local read "Static output"() -> (w411:T2)
                n62 = local read "GPIB output"() -> (w410:T1)
                n63 = local read "Output Data"() -> (w412:i64[][])
                n64 = local write "GPIB temp"(w410) -> ()
                n65 = local write "Static temp"(w411) -> ()
                n66 = local write "Temp"(w412) -> ()
              }
            }
          }
        }
        "Numeric" <- w24
      }
    }
    frame #1 {
      # "This sequence frame takes care of triggering the static DAQ's initial and final voltages. The DAQ card\nstrangely outputs the first entry in a voltage array immediately after being programmed. So, the \nsolution was to pad the voltage array with the default voltages as the initial voltages."
    }
  }
  "Output Data" <- w1
  "Static output" <- w5
  "GPIB output" <- w3
  "Temp" <- w6
  "Static temp" <- w7
  "GPIB temp" <- w4
